vi "PortCullis.vi"(6 "Extra_Dist":dbl, 7 "Level":bool, 8 "Auto_Enable":bool=TRUE, 9 "Auto_Selection":T1=enum."Cheval de Frise", 10 "Yaw":dbl=-4.802742406845094, 11 "Encoder":dbl=185.13304649999998) -> (0 "Rest_Encoder":bool, 1 "Intake Arm Lowered":bool, 2 "PortCullis_Enable":bool, 3 "Motor Speed":dbl, 4 "Completed_Auto":bool, 5 "Rest_Gyro":bool)   [LabVIEW 2015]
uses:
  Auto_Selection.ctl
  AutoEnum.ctl
  <vilib>/Rock Robotics/Network Tables/NT Read Number.vi
panel:
  in  "DB_Count":dbl=3.0
  in  "Drive_Speed":dbl=-1.0 format="%#_13g"
  in  "Distance Stop":dbl=180.0
  in  "Clear Error":bool
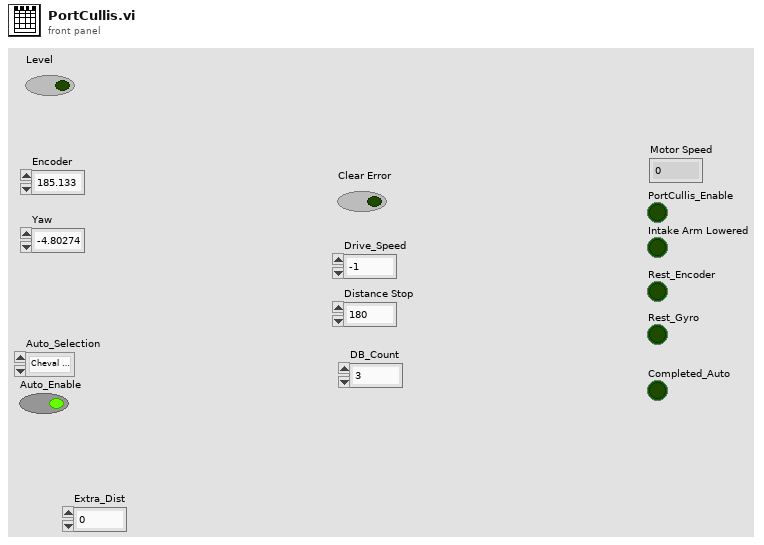
[diagram p1: front panel]
types:
  T1 = typedef "Auto_Selection.ctl" = enum16{"Low Bar", "Rough Terrain", "Rock Wall", "Ramparts", "Moat", "Cheval de Frise", "Portcullis", "None", "One  Ball", "Shoot"}
  T2 = typedef "AutoEnum.ctl" = enum16{"Off", "ResetVar", "ResetOff", "BeforeTeeter", "LowerArm", "DriveForward", "Stop", "Stop One", "Drive Back", "Drive Forward Two"}
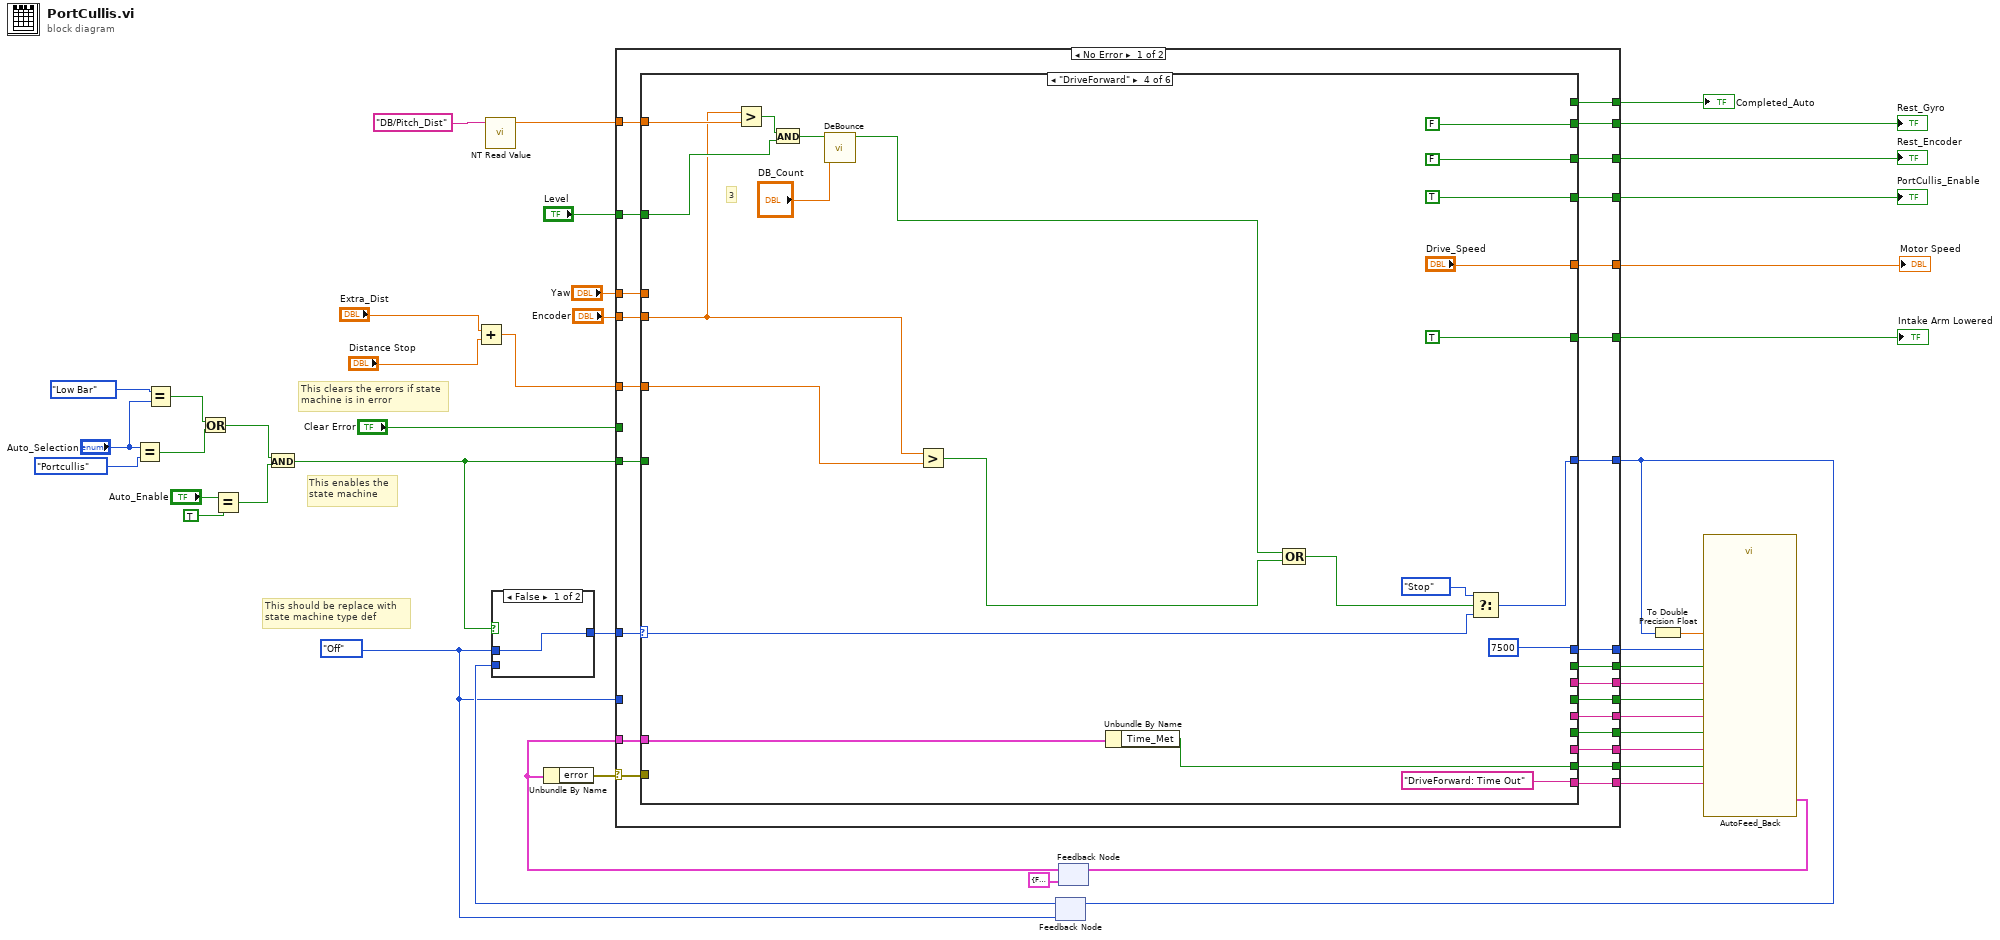
[diagram p0: block diagram]
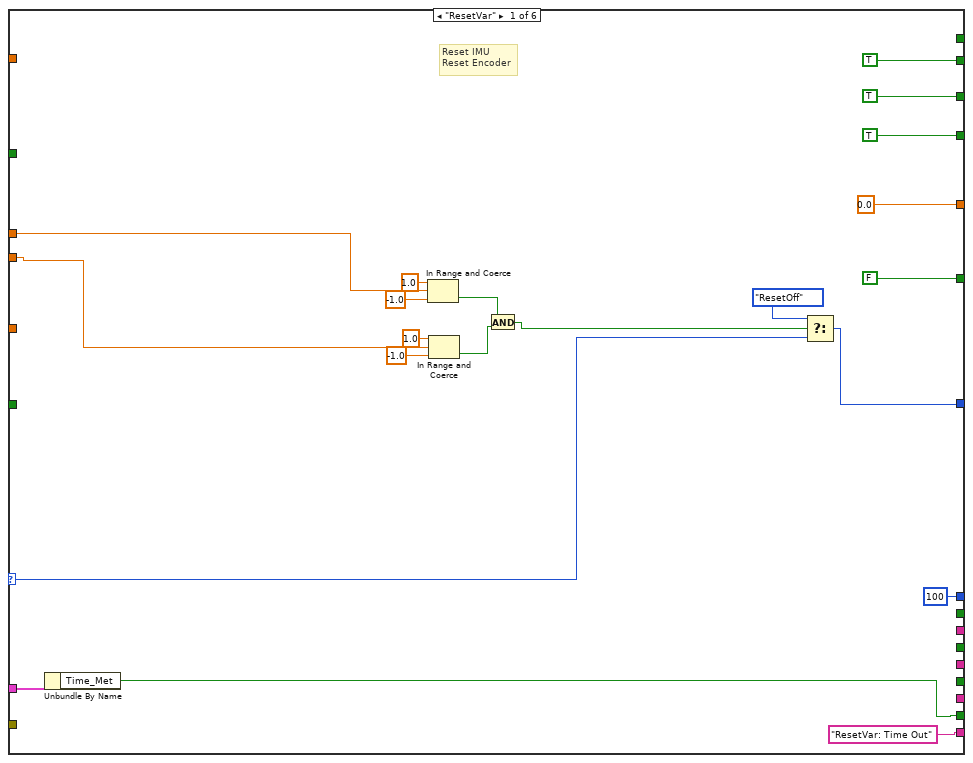
[diagram p3: hidden frame]
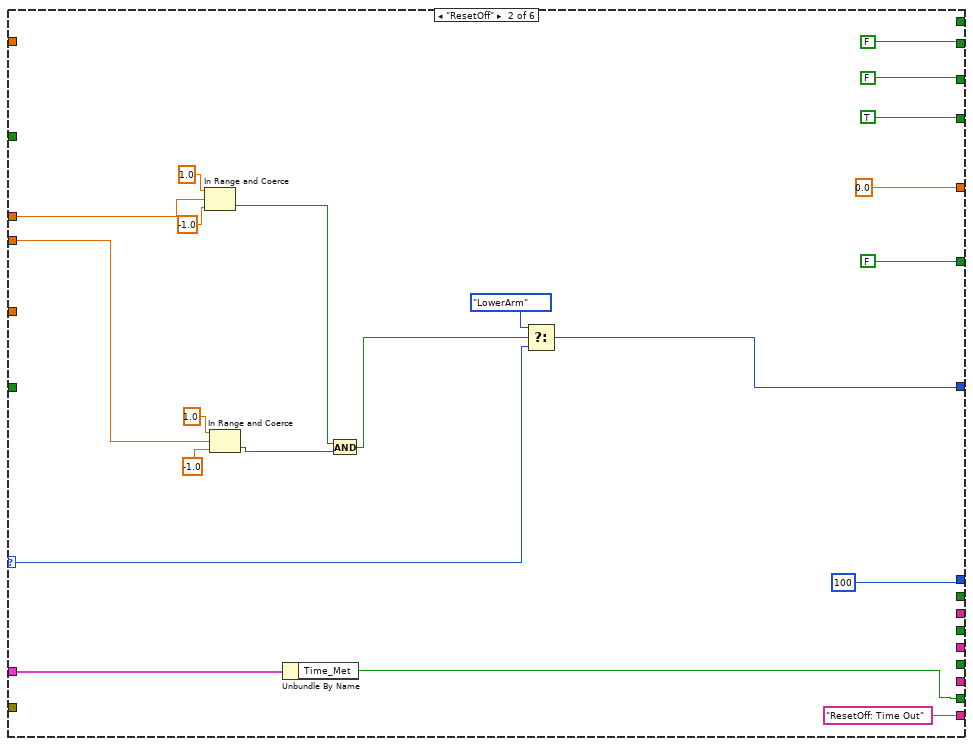
[diagram p4: hidden frame]
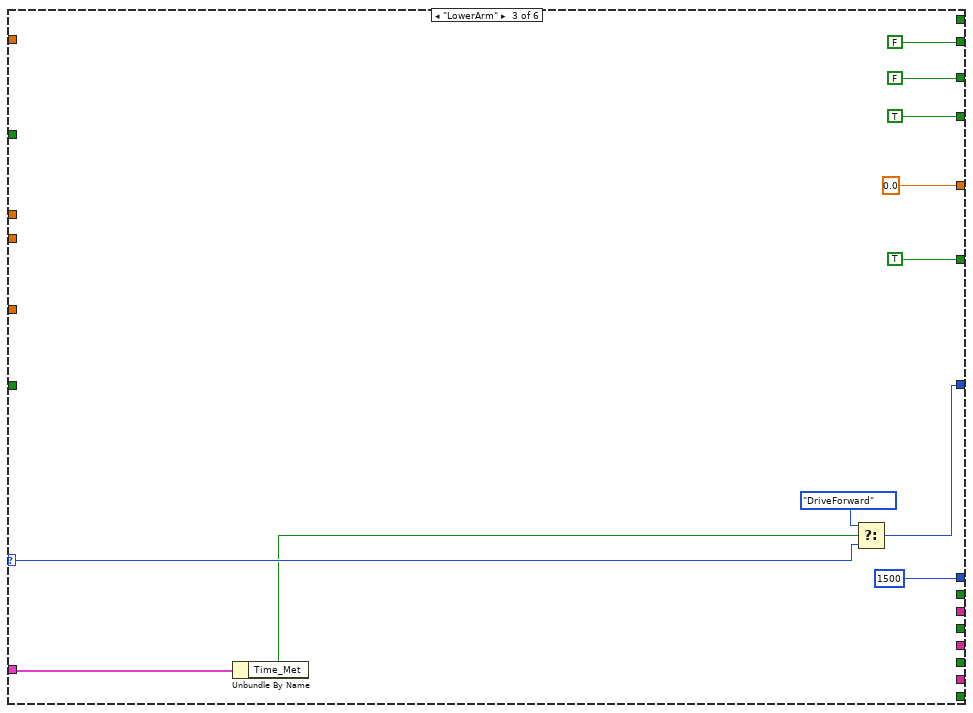
[diagram p5: hidden frame]
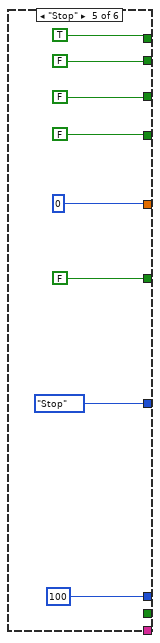
[diagram p6: hidden frame]
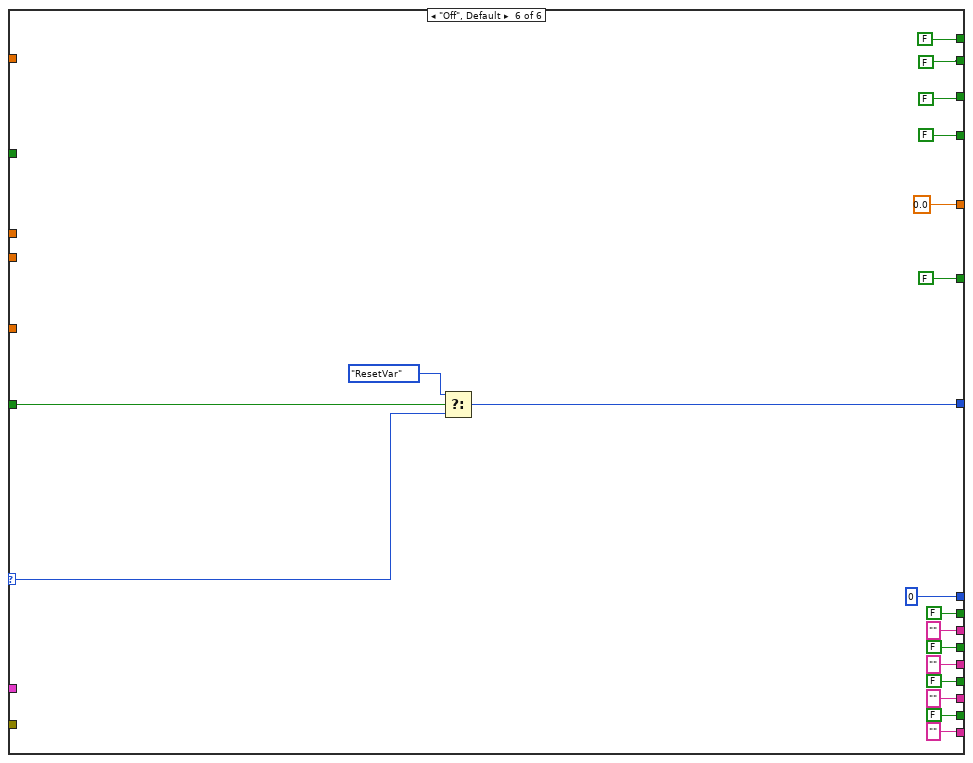
[diagram p7: hidden frame]
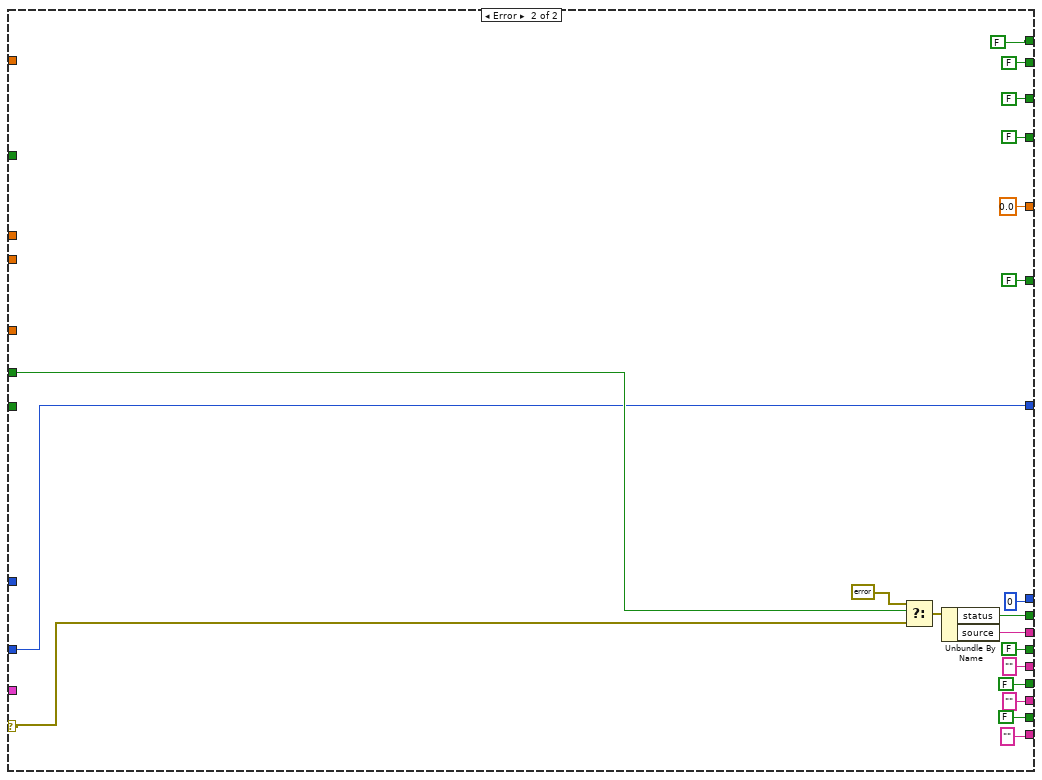
[diagram p8: hidden frame]
diagram:
  w32 = AutoEnum."Off"
  # "This clears the errors if state \nmachine is in error"
  # "This enables the \nstate machine"
  # "This should be replace with \nstate machine type def"
  n1 = Equal?(x="Auto_Selection", y=Auto_Selection."Portcullis" ("Auto_Selection 2")) -> (x = y?=w9:bool)
  n2 = Equal?(x=Auto_Selection."Low Bar" ("Auto_Selection 2"), y="Auto_Selection") -> (x = y?=w10:bool)
  n3 = Or(x=w10, y=w9) -> (x .or. y?=w8:bool)
  n4 = Equal?(x="Auto_Enable", y=TRUE) -> (x = y?=w22:bool)
  n5 = And(x=w8, y=w22) -> (x .and. y?=w21:bool)
  n6 = Add(x="Extra_Dist", y="Distance Stop") -> (x+y=w4:dbl)
  n7 = call-poly <vilib>:"NT Read Value.vi"("Name"="DB/Pitch_Dist" ("refnum name")) -> ("Numeric"=w1:dbl)  [unwired: 9 in, 1 out]
  n8 = feedback #1(w32) -> (w34:T2)
  n9 = case shown="False" w21 {
    tunnel: w32 -> [w44 _]
    tunnel: [w44 w45] -> w35
    tunnel: w34 -> [_ w45]
    frame False {
    }
    frame True {
    }
  }
  n10 = feedback #2(cluster{"Time_Met":bool, "error ":errorcluster} {"Time_Met"=FALSE, "error "={"status"=FALSE, "code"=0, "source"=""}} ("Feedback_State")) -> (w36:cluster{"Time_Met":bool, "error ":errorcluster})
  n11 = Unbundle By Name(w36) -> ("error"=w38:errorcluster)
  n12 = case shown="No Error" w38 {
    selector: w38 -> [w65 w189]
    tunnel: [w70 FALSE] -> w43
    tunnel: [w69 FALSE] -> w42
    tunnel: [w68 w186] -> w26
    tunnel: [w67 0] -> w41
    tunnel: "Clear Error" -> [_ w188]
    tunnel: w36 -> [w66 _]
    tunnel: w21 -> [w64 _]
    tunnel: w35 -> [w63 _]
    tunnel: w32 -> [_ w186]
    tunnel: [w62 0.0] -> w31
    tunnel: [w61 FALSE] -> w30
    tunnel: [w60 FALSE] -> w29
    tunnel: "Yaw" -> [w59 _]
    tunnel: "Encoder" -> [w58 _]
    tunnel: [w57 w181] -> w20
    tunnel: [w56 w180] -> w19
    tunnel: [w55 FALSE] -> w18
    tunnel: [w54 ""] -> w17
    tunnel: [w53 FALSE] -> w16
    tunnel: [w52 ""] -> w15
    tunnel: [w51 FALSE] -> w14
    tunnel: [w50 ""] -> w13
    tunnel: [w49 FALSE] -> w7
    tunnel: w4 -> [w48 _]
    tunnel: "Level" -> [w47 _]
    tunnel: w1 -> [w46 _]
    frame No Error {
      n13 = case shown="\"DriveForward\"" w63 {
        selector: w63 -> [w82 w94 w115 w139 _ w168]
        tunnel: [TRUE FALSE FALSE FALSE FALSE FALSE] -> w70
        tunnel: [TRUE FALSE FALSE FALSE FALSE FALSE] -> w69
        tunnel: [100 100 1500 7500 100 0] -> w67
        tunnel: [w83 w95 w114 w138 AutoEnum."Stop" w167] -> w68
        tunnel: w66 -> [w90 w107 w118 w143 _ _]
        tunnel: w65 -> [_ _ _ _ _ _]
        tunnel: w64 -> [_ _ _ _ _ w169]
        tunnel: [0.0 0.0 0.0 "Drive_Speed" 0 0.0] -> w62
        tunnel: [TRUE TRUE TRUE TRUE FALSE FALSE] -> w61
        tunnel: [FALSE FALSE TRUE TRUE FALSE FALSE] -> w60
        tunnel: w59 -> [w76 w96 _ _ _ _]
        tunnel: w58 -> [w75 w97 _ w124 _ _]
        tunnel: [_ _ _ _ _ FALSE] -> w57
        tunnel: [_ _ _ _ _ ""] -> w56
        tunnel: [_ _ _ _ _ FALSE] -> w55
        tunnel: [_ _ _ _ _ ""] -> w54
        tunnel: [_ _ _ _ _ FALSE] -> w53
        tunnel: [_ _ _ _ _ ""] -> w52
        tunnel: [w79 w92 _ w135 _ FALSE] -> w51
        tunnel: ["ResetVar: Time Out" ("source") "ResetOff: Time Out" ("source") _ "DriveForward: Time Out" ("source") _ ""] -> w50
        tunnel: [_ _ _ _ TRUE FALSE] -> w49
        tunnel: w48 -> [_ _ _ w133 _ _]
        tunnel: w47 -> [_ _ _ w127 _ _]
        tunnel: w46 -> [_ _ _ w125 _ _]
        frame "ResetVar" {
          # "Reset IMU\nReset Encoder"
          n14 = Unbundle By Name(w90) -> ("Time_Met"=w79:bool)
          n15 = In Range and Coerce(upper limit=1.0, x=w76, lower limit=-1.0) -> (In Range?=w78:bool)  [unwired: 1 out]
          n16 = In Range and Coerce(upper limit=1.0, x=w75, lower limit=-1.0) -> (In Range?=w77:bool)  [unwired: 1 out]
          n17 = And(x=w78, y=w77) -> (x .and. y?=w84:bool)
          n18 = Select(t=AutoEnum."ResetOff", s=w84, f=w82) -> (s? t:f=w83:T2)
        }
        frame "ResetOff" {
          n19 = In Range and Coerce(upper limit=1.0, x=w96, lower limit=-1.0) -> (In Range?=w103:bool)  [unwired: 1 out]
          n20 = In Range and Coerce(upper limit=1.0, x=w97, lower limit=-1.0) -> (In Range?=w101:bool)  [unwired: 1 out]
          n21 = Unbundle By Name(w107) -> ("Time_Met"=w92:bool)
          n22 = And(x=w103, y=w101) -> (x .and. y?=w98:bool)
          n23 = Select(t=AutoEnum."LowerArm", s=w98, f=w94) -> (s? t:f=w95:T2)
        }
        frame "LowerArm" {
          n24 = Unbundle By Name(w118) -> ("Time_Met"=w113:bool)
          n25 = Select(t=AutoEnum."DriveForward", s=w113, f=w115) -> (s? t:f=w114:T2)
        }
        frame "DriveForward" {
          # "3"
          n26 = Greater?(x=w124, y=w125) -> (0:w130:bool)
          n27 = And(x=w130, y=w127) -> (x .and. y?=w129:bool)
          n28 = call "DeBounce.vi"("DB_Count"="DB_Count", "Value"=w129) -> ("BD_Value"=w126:bool)  [unwired: 9 in]
          n29 = Greater?(x=w124, y=w133) -> (0:w132:bool)
          n30 = Unbundle By Name(w143) -> ("Time_Met"=w135:bool)
          n31 = Compound Arithmetic op=OR(w126, w132) -> (w131:bool)
          n32 = Select(t=AutoEnum."Stop", s=w131, f=w139) -> (s? t:f=w138:T2)
        }
        frame "Stop" {
        }
        frame "Off", Default {
          n33 = Select(t=AutoEnum."ResetVar", s=w169, f=w168) -> (s? t:f=w167:T2)
        }
      }
    }
    frame Error {
      n34 = Select(t=errorcluster {"status"=FALSE, "code"=0, "source"=""}, s=w188, f=w189) -> (s? t:f=w182:errorcluster)
      n35 = Unbundle By Name(w182) -> ("status"=w181:bool, "source"=w180:string)
    }
  }
  "Rest_Gyro" <- w43
  "Rest_Encoder" <- w42
  "Motor Speed" <- w31
  "PortCullis_Enable" <- w30
  "Intake Arm Lowered" <- w29
  "Completed_Auto" <- w7
  n36 = feedback-in #1(w26) -> ()
  n37 = To Double Precision Float(number=w26) -> (double precision float=w33:dbl)
  n38 = call "AutoFeed_Back.vi"("Code 4"=w13, "Error_4_En"=w14, "Code 3"=w15, "Code 2"=w17, "Error_3_En"=w16, "Error_2_En"=w18, "Code 1"=w19, "Error_1_En"=w20, "Time (ms)"=w41, "State"=w33) -> ("Feedback_State"=w40:cluster{"Time_Met":bool, "error ":errorcluster})  [unwired: 1 in]
  n39 = feedback-in #2(w40) -> ()
